vi "iDDS to FPGA.vi"(11 "Chirp Parameters":T1 {"miniscantime" format="%#_6e"}) -> (1 "HEX Array":string[](array[string]), 3 "Interrupted":bool)   [LabVIEW 2013]
uses:
  Controls/Chirp Parameters.ctl
  Controls/Frequency Record.ctl
  Controls/Amplitude Record.ctl
  Typedefs/HW config states enum.ctl
  Global Variables/General Globals.vi
panel:
  out "Loop index":i32
  # "RE-ENTRANT"
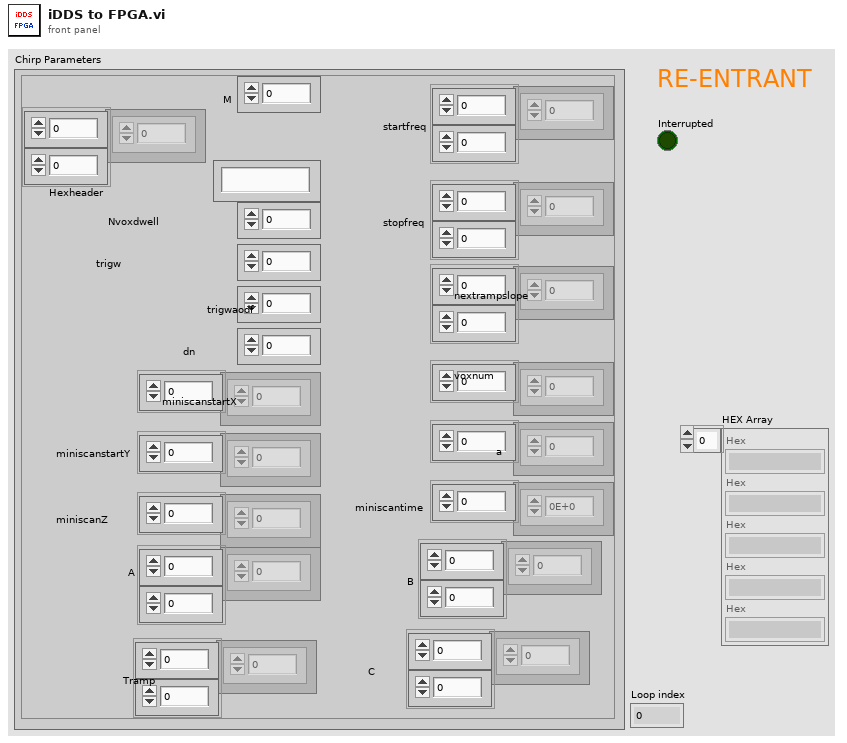
[diagram p1: front panel]
types:
  T1 = typedef "Chirp Parameters.ctl" = cluster{"M":dbl, "miniscantime":dbl[], "startfreq":dbl[][], "stopfreq":dbl[][], "nextrampslope":dbl[][], "Hexheader":string, "voxnum":dbl[], "Nvoxdwell":dbl, "miniscanstartX":dbl[], "miniscanstartY":dbl[], "miniscanZ":dbl[], "trigw":dbl, "trigwaodf":dbl, "dn":dbl, "a":dbl[], "A":dbl[][], "B":dbl[][], "Tramp":dbl[][], "C":dbl[][], "Amplitude":dbl[][]}
  T2 = typedef "HW config states enum.ctl" = enum16{"Load from file", "Save to file", "Write all", "Read all", "Write XY stage settings", "Write DAQ FPGA settings", "Write Control FPGA settings", "Write Phys Channels", "Clear", "Compare from file"}
  T3 = typedef "Amplitude Record.ctl" = cluster{"A":dbl[], "Mu":dbl[], "Sigma":dbl[], "IGD":dbl[], "N":dbl[]}
  T4 = typedef "Frequency Record.ctl" = cluster{"Phi":dbl[], "A":dbl[], "B":dbl[], "C":dbl[], "D":dbl[], "E":dbl[], "Tstart":dbl[], "Tframe":dbl[]}
  T5 = typedef "Sys Configuration.ctl" = cluster{"XY Stage":T6, "DAQ FPGA":T7, "Control system":T11, "Encoder":T12, "DAQmx Chan":T13, "Computer MAC address":string, "Cam VidRec":T14, "Externalise Triggers":bool, "Laser wavelength (nm)":dbl}
  T6 = typedef "XY Stage config cluster.ctl" = cluster{"COM port":refnum<visa-resource-name>, "XY stage available":bool}
  T7 = typedef "DAQ FPGA config cluster.ctl" = cluster{"Ref":T8, "Target":T9, "Clock Freq (MHz) ":dbl, "input card type":T10, "Samples Wait after Trigger":u16, "AOD fill":u16, "StartupDelay":i32, "Slip Cycle (clock cycles)":u32, "Add Cycle":bool}
  T8 = typedef "FPGA Ref.ctl" = refnum<k20>
  T9 = typedef "nirio_resource_hc.ctl" = tag
  T10 = typedef "FPGA input type AC-DC.ctl" = enum16{"AC Card", "DC Card"}
  T11 = typedef "CTRL system config cluster.ctl" = cluster{"Ethernet opened":bool, "Ethernet Port":u32, "Ctrl FPGA available":bool, "Ctrl FPGA Clock (MHz)":dbl, "Ctrl system MAC address":string, "Control system.Network adapter name":string, "AOD 1 Amplitude":i16, "AOD 2 Amplitude":i16, "AOD 3 Amplitude":i16, "AOD 4 Amplitude":i16, "Data Time Interval (ns)":dbl, "T0 (ns)":dbl, "Ta (ns)":dbl}
  T12 = typedef "Encoder config cluster.ctl" = cluster{"IP address":string, "Port":u16, "Encoder available":bool, "Wheel radius (cm)":dbl}
  T13 = typedef "DAQmx physical channels cluster.ctl" = cluster{"Pockels AO":tag, "Hard shutter AO":tag, "PMT AOs":tag, "Power meter AI":tag}
  T14 = typedef "Cam VidRec HW config setup cluster.ctl" = cluster{"DO flag-Video record":tag, "DO flag-Trial start":tag, "VidRec available":bool}
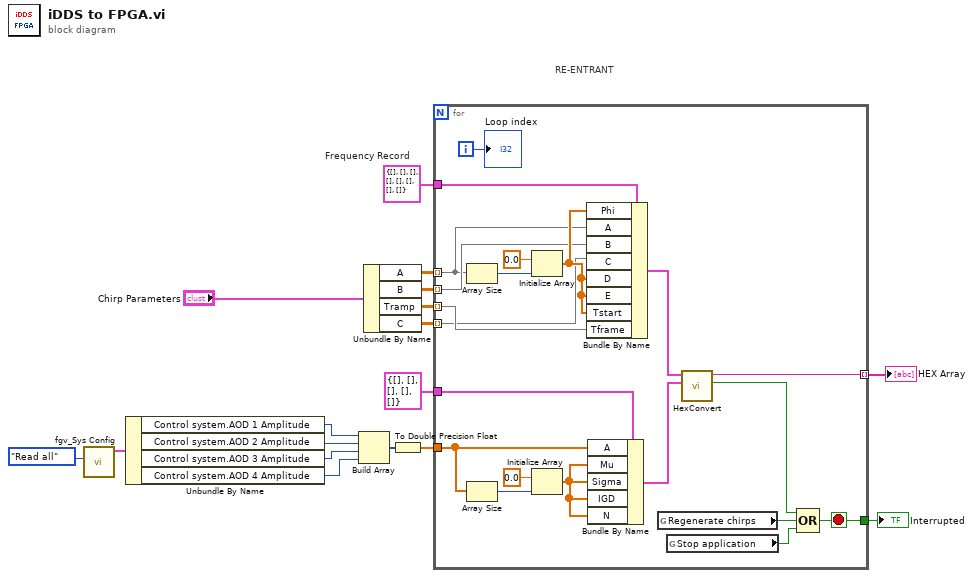
[diagram p0: block diagram]
diagram:
  w17 = T4 {"Phi"=[], "A"=[], "B"=[], "C"=[], "D"=[], "E"=[], "Tstart"=[], "Tframe"=[]}  # Frequency Record
  # "RE-ENTRANT"
  n1 = call "fgv_Sys Config.vi"("Function"=HW_config_states_enum."Read all") -> ("System Config out"=w2:T5)  [unwired: 9 in, 1 out]
  n2 = Unbundle By Name(w2) -> ("Control system.AOD 1 Amplitude"=w13:i16, "Control system.AOD 2 Amplitude"=w12:i16, "Control system.AOD 3 Amplitude"=w11:i16, "Control system.AOD 4 Amplitude"=w10:i16)
  n3 = Build Array(w13, w12, w11, w10) -> (w8:i16[])
  n4 = Unbundle By Name("Chirp Parameters") -> ("A"=w9:dbl[][], "B"=w6:dbl[][], "Tramp"=w7:dbl[][], "C"=w5:dbl[][])
  n5 = To Double Precision Float(number=w8) -> (double precision float=w1:dbl[])
  n6 = for {
    tunnel: w9 -> [w26] mode=indexing
    tunnel: w17 -> [w34]
    tunnel: T3 {"A"=[], "Mu"=[], "Sigma"=[], "IGD"=[], "N"=[]} ("Amplitude Record") -> [w33]
    tunnel: w1 -> [w29]
    tunnel: w7 -> [w25] mode=indexing
    tunnel: w6 -> [w27] mode=indexing
    tunnel: w5 -> [w24] mode=indexing
    tunnel: [w21] -> w14 mode=indexing
    tunnel: [w20] -> w4
    i -> [w28]
    stop <- w20 stop-if-true
    n7 = Array Size(array=w26) -> (size(s)=w36:i32)
    n8 = Array Size(array=w29) -> (size(s)=w32:i32)
    n9 = Initialize Array(0.0 ("element"), w36) -> (w35:dbl[])
    n10 = Initialize Array(0.0 ("element"), w32) -> (w30:dbl[])
    n11 = Bundle By Name(cluster=w34, "Phi"=w35, "A"=w26, "B"=w27, "C"=w24, "D"=w35, "E"=w35, "Tstart"=w35, "Tframe"=w25) -> (w23:T4)
    n12 = Bundle By Name(cluster=w33, "A"=w29, "Mu"=w30, "Sigma"=w30, "IGD"=w30, "N"=w30) -> (w22:T3)
    n13 = global read "General Globals.vi" "Regenerate chirps"() -> (w20:bool)
    n14 = global read "General Globals.vi" "Stop application"() -> (w18:bool)
    n15 = call "HexConvert.vi"("Amplitude Record"=w22, "Frequency Record"=w23) -> ("Interrupted"=w19:bool, "Hex"=w21:string)  [unwired: 8 in]
    n16 = Compound Arithmetic op=OR(w19, w20, w18) -> ()  [unwired: 1 out]
    "Loop index" <- w28
  }
  "HEX Array" <- w14
  "Interrupted" <- w4
